vi "disable pre-execution timing reporting.vi"(8 "error in":errorcluster, 11 "Standard Engine Configuration in":refnum<class "Standard Engine Configuration.lvclass">) -> (0 "error out":errorcluster, 3 "Standard Engine Configuration out":refnum<class "Standard Engine Configuration.lvclass">)   [LabVIEW 2013, in "Standard Engine Configuration.lvclass"]
doc: "Disables the timing reporting if enabled by the 'enable timing reporting.vi'."
uses:
  Standard Engine Configuration.lvclass
  <vilib>/NI/Configuration Framework/serializable configuration/NISE_CEF_serializable configuration.lvclass/NISE_CEF_serializable configuration.ctl
  Standard Engine Configuration.lvclass/Standard Engine Configuration.ctl
  execution timing tags.ctl
  <vilib>/Utility/LVClass/Get LV Class Name.vi
  <vilib>/NI/Configuration Framework/error generator/NISE_error generator.vi
  <vilib>/NI/Module Execution Interface/Engine Configuration/engine configuration.lvclass
  <vilib>/NI/Configuration Framework/serializable configuration/NISE_CEF_serializable configuration.lvclass
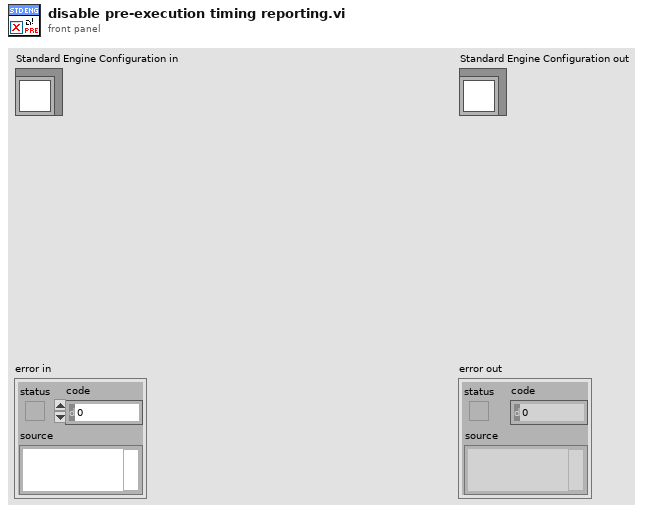
[diagram p1: front panel]
types:
  T1 = typedef "Standard Engine Configuration.lvclass/execution timing tags.ctl" = cluster{"iteration start time (DBL)":string, "post inputs time (DBL)":string, "post process time (DBL)":string, "post outputs time (DBL)":string}
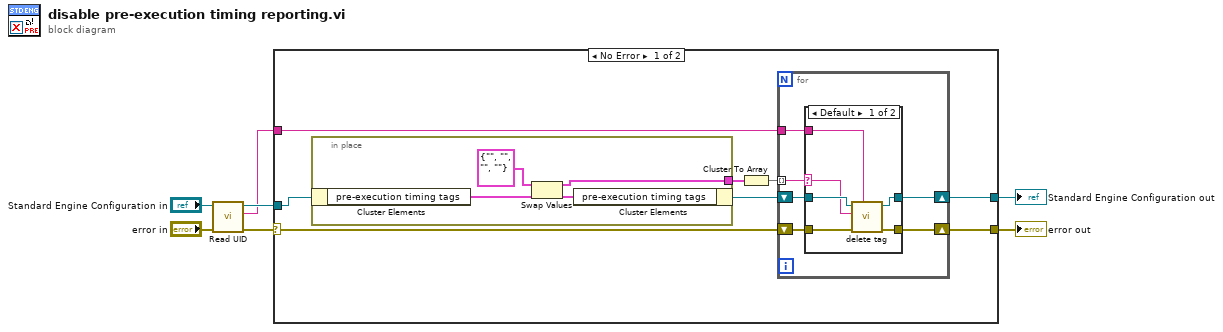
[diagram p0: block diagram]
diagram:
  n1 = call <vilib>:"Read UID.vi"("error in"="error in", "configuration in"="Standard Engine Configuration in") -> ("error out"=w1:errorcluster, "instance id"=w3:string, "configuration out"=w6:refnum<class "Standard Engine Configuration.lvclass">)  [unwired: 7 in]
  n2 = case shown="No Error" w1 {
    selector: w1 -> [w12 w35]
    tunnel: [w11 w35] -> w5
    tunnel: w6 -> [w15 w34]
    tunnel: [w13 w34] -> w4
    tunnel: w3 -> [w9 _]
    frame No Error {
      n3 = in-place {
        in-place-border: [w31] -> w8
        n4 = in-place-cluster #1(w15) -> ("pre-execution timing tags"=w33:T1)
        n5 = Swap Values(12:T1 {"iteration start time (DBL)"="", "post inputs time (DBL)"="", "post process time (DBL)"="", "post outputs time (DBL)"=""} ("pre-execution timing tags"), 14:w33) -> (1:w31:T1, 3:w32:T1)  [unwired: 1 in]
        n6 = in-place-cluster #1("pre-execution timing tags"=w32) -> (w14:refnum<class "Standard Engine Configuration.lvclass">)
      }
      n7 = Cluster To Array(cluster=w8) -> (array=w10:string[])
      n8 = for {
        shift-right: [w21] -> w13
        shift-left: w14 -> [w20]
        shift-right: [w18] -> w11
        shift-left: w12 -> [w19]
        tunnel: w10 -> [w16] mode=indexing
        tunnel: w9 -> [w17]
        n9 = case shown="Default" w16 {
          selector: w16 -> [w26 _]
          tunnel: [w23 w29] -> w21
          tunnel: w20 -> [w27 w29]
          tunnel: w19 -> [w25 w28]
          tunnel: [w24 w28] -> w18
          tunnel: w17 -> [w22 _]
          frame Default {
            n10 = call <vilib>:"delete tag.vi"("owner ID"=w22, "error in"=w25, "tag name"=w26, "engine configuration in"=w27) -> ("error out"=w24:errorcluster, "engine configuration out"=w23:refnum<class "Standard Engine Configuration.lvclass">)  [unwired: 6 in]
          }
          frame "" {
          }
        }
      }
    }
    frame Error {
      # "delete any new tags if any fails"
    }
  }
  "error out" <- w5
  "Standard Engine Configuration out" <- w4
